vi "IR Voltage To Distance.vi"(5 "IR Voltage":dbl) -> (2 "Distance (0-100)":dbl)   [LabVIEW 2014]
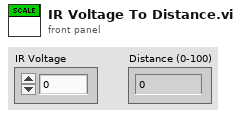
[diagram p1: front panel]
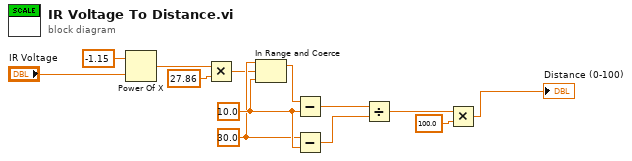
[diagram p0: block diagram]
diagram:
  w10 = 10.0 ("upper limit 2")
  w9 = 30.0 ("upper limit")
  n1 = Power Of X(1:"IR Voltage", 2:-1.15 ("x")) -> (0:w2:dbl)
  n2 = Multiply(x=w2, y=27.86 ("y 5")) -> (x*y=w4:dbl)
  n3 = In Range and Coerce(upper limit=w9, x=w4, lower limit=w10) -> (coerced(x)=w5:dbl)  [unwired: 1 out]
  n4 = Subtract(x=w5, y=w10) -> (x-y=w6:dbl)
  n5 = Subtract ("Subtract 2")(x=w9, y=w10) -> (x-y=w11:dbl)
  n6 = Divide ("Divide 2")(x=w6, y=w11) -> (x/y=w7:dbl)
  n7 = Multiply ("Multiply 2")(x=w7, y=100.0 ("y 6")) -> (x*y=→"Distance (0-100)":dbl)
